vi "onInterrupt.vi"(8 "error in (no error)":errorcluster, 11 "ContextThisComponent in":refnum<class "ContextThisComponent.lvclass">) -> (0 "error out":errorcluster, 3 "ContextThisComponent out":refnum<class "ContextThisComponent.lvclass">)   [LabVIEW 2012, in "ContextThisComponent.lvclass"]
uses:
  ContextThisComponent.lvclass
  ContextThisComponent.lvclass/ContextThisComponent.ctl
  IStateFactory/IStateFactory.lvclass
  IModel/IModel.lvclass
  State/State.lvclass
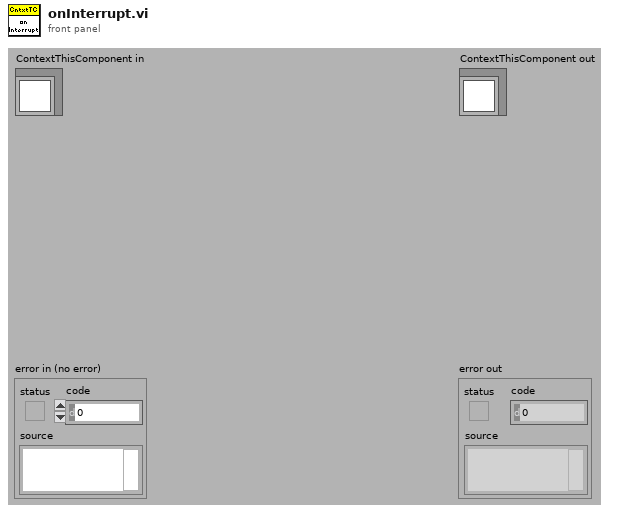
[diagram p1: front panel]
types:
  T1 = typedef "EXATypedefs.lvlib/StateValue.ctl" = enum16{"DisabledState", "EnabledState", "FaultState", "OffState", "StandbyState"}
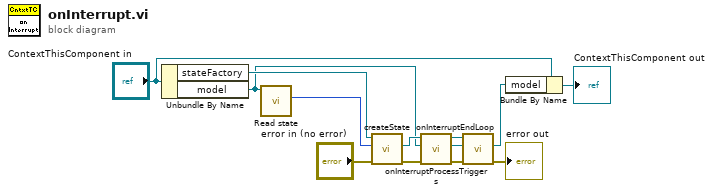
[diagram p0: block diagram]
diagram:
  n1 = Unbundle By Name("ContextThisComponent in") -> ("stateFactory"=w10:refnum<class "IStateFactory.lvclass">, "model"=w7:refnum<class "IModel.lvclass">)
  n2 = call-dynamic "Read state.vi"("IModel in"=w7) -> ("StateValue"=w9:T1)  [unwired: 9 in, 1 out]
  n3 = call-dynamic "createState.vi"("error in (no error)"="error in (no error)", "stateValue"=w9, "IStateFactory in"=w10) -> ("error out"=w6:errorcluster, "state"=w8:refnum<class "State.lvclass">)  [unwired: 6 in, 1 out]
  n4 = call-dynamic "onInterruptProcessTriggers.vi"("error in (no error)"=w6, "model in"=w7, "State in"=w8) -> ("error out"=w3:errorcluster, "model out"=w4:refnum<class "IModel.lvclass">, "State out"=w5:refnum<class "State.lvclass">)  [unwired: 6 in]
  n5 = call-dynamic "onInterruptEndLoop.vi"("error in (no error)"=w3, "model in"=w4, "State in"=w5) -> ("error out"=→"error out":errorcluster, "model out"=w1:refnum<class "IModel.lvclass">)  [unwired: 6 in, 1 out]
  n6 = Bundle By Name(cluster="ContextThisComponent in", "model"=w1) -> (→"ContextThisComponent out":refnum<class "ContextThisComponent.lvclass">)
